vi "Palette Visibility.vi"(8 "error in (no error)":errorcluster, 9 "Clust Refnum":refnum<vi>, 10 "IntGraph Refnum":refnum<vi>, 11 "Visible?":bool) -> (0 "error out":errorcluster)   [LabVIEW 2020, in "3D Plot.lvclass"]
uses:
  <vilib>/Math Plots/3D Math Plots/3D Plot/3D Plot/3D Plot.lvclass
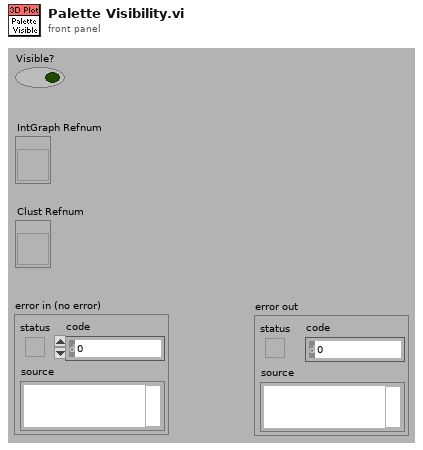
[diagram p1: front panel]
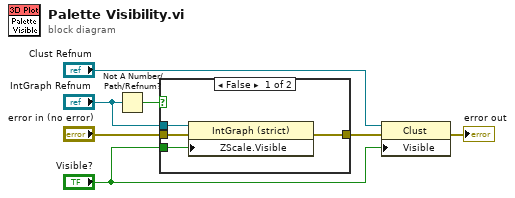
[diagram p0: block diagram]
diagram:
  n1 = Not A Number/Path/Refnum?(number/path/refnum="IntGraph Refnum") -> (NaN/Path/Refnum?=w1:bool)
  n2 = case shown="False" w1 {
    tunnel: "Visible?" -> [w8 _]
    tunnel: [w11 w12] -> w5
    tunnel: "error in (no error)" -> [w10 w12]
    tunnel: "IntGraph Refnum" -> [w9 _]
    frame False {
      n3 = property on="Property Node" class="IntGraph (strict)"(reference=w9, error in=w10, "ZScale.Visible"=w8) -> (error out=w11:errorcluster)  [unwired: 1 out]
    }
    frame True {
    }
  }
  n4 = property on="Property Node" class="Clust"(reference="Clust Refnum", error in=w5, "Visible"="Visible?") -> (error out=→"error out":errorcluster)  [unwired: 1 out]
